vi "RIB - eSTOP 1.vi"(0 "Limits File Path":path, 5 "Results File Path":path, 11 "error in":errorcluster) -> (15 "error out":errorcluster)   [LabVIEW 2024]
doc: "Template test"
uses:
  <vilib>/addons/_JKI Toolkits/State Machine/_JKI_lib_State_Machine.llb/Select State(s)_err__jki_lib_state_machine.vi
  <vilib>/addons/_JKI Toolkits/State Machine/_JKI_lib_State_Machine.llb/Select State(s)_bool__jki_lib_state_machine.vi
  <vilib>/addons/_JKI Toolkits/State Machine/_JKI_lib_State_Machine.llb/Periodic Trigger__ogtk__JKI-SM__jki_lib_state_machine.vi
  <userlib>/_OpenG.lib/file/file.llb/Strip Path Extension - String__ogtk.vi
  <vilib>/Utility/file.llb/Read Delimited Spreadsheet (string).vi
  <userlib>/_OpenG.lib/file/file.llb/openg_file.lvlib
  <userlib>/_OpenG.lib/appcontrol/appcontrol.llb/openg_application_control.lvlib
  <userlib>/_OpenG.lib/time/time.llb/openg_time.lvlib
  <vilib>/Utility/file.llb/Write Delimited Spreadsheet (string).vi
panel:
  out "UDP Read Bar 2":dbl(slide) scale=0.0..10.0
  out "UDP Read Bar":dbl(slide) scale=0.0..10.0
  out "eSTOP 1 Test":bool
  out "eSTOP 1 Error Test":bool
  in  "eSTOP 1 Error Test":string
  in  "eSTOP 1 Test":string
  in  "connection ID":refnum<k16>
  out "Results Data Array":string[][](array[string])
  in  "handle out":u64
  in  "Exit":bool
  # "eSTOP 1 Test"
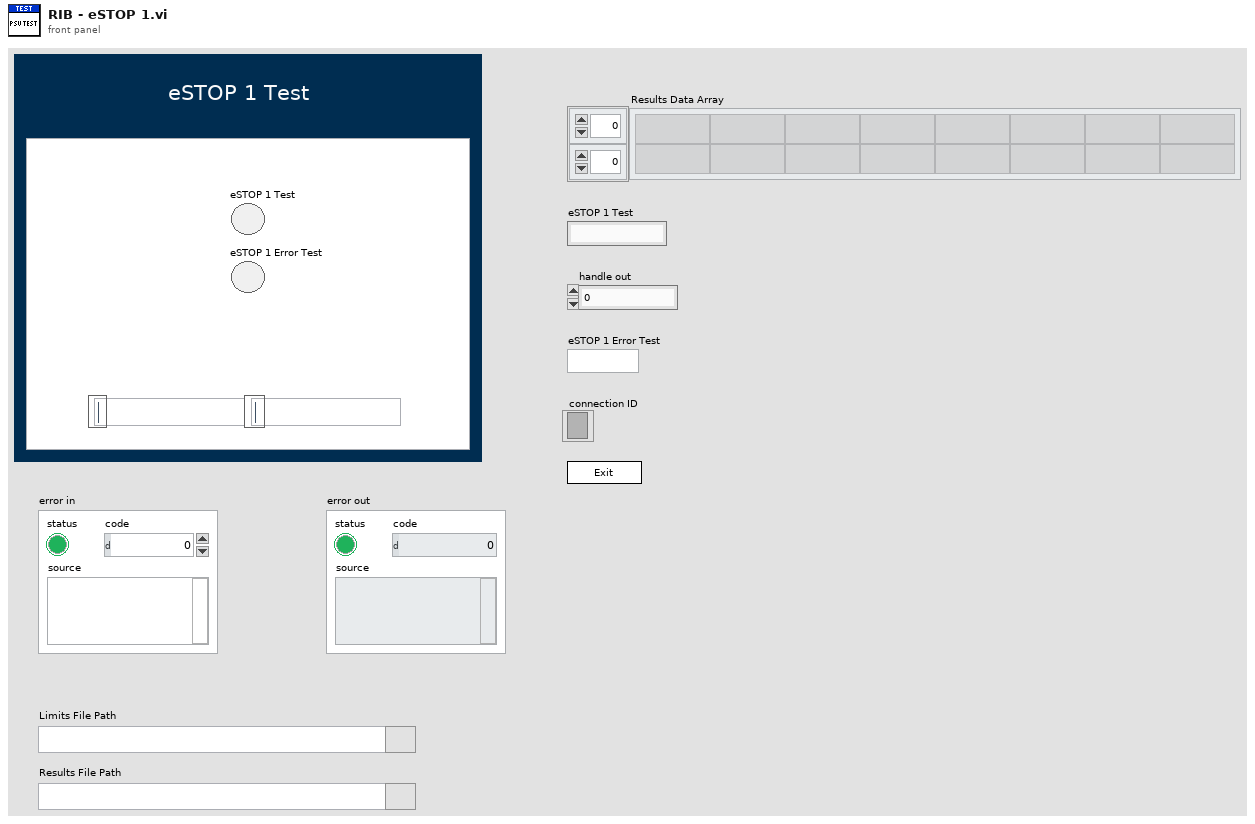
[diagram p1: front panel]
types:
  T1 = enum32{"Invalid", "Standard", "Closed", "Hidden", "Minimized", "Maximized"}
  T2 = enum32{"invalid app kind", "Development System", "Run Time System", "Student Edition", "Embedded LabVIEW", "Evaluation", "Custom"}
  T3 = typedef "FGV - Enum" = enum16{"Cleanup", "Get Data", "Open UDP", "Initialise DAQ", "Initialise I2C"}
  T4 = enum16{"Start Timer", "Get Time", "Pause", "Unpause"}
  T5 = cluster{"Core":cluster{"Current VI Reference":refnum<vi>, "Close Panel on Exit?":bool}, "Limits File Path":path, "Test Limits":string[][], "Results Data Array":string[][], "Results File Path":path, "Voltage":dbl, "connection ID":refnum<k16>, "handle out":u64, "eSTOP 1 Test":string, "eSTOP 1 Error Test":string}
  T6 = cluster{"Current VI Reference":refnum<vi>, "Close Panel on Exit?":bool}
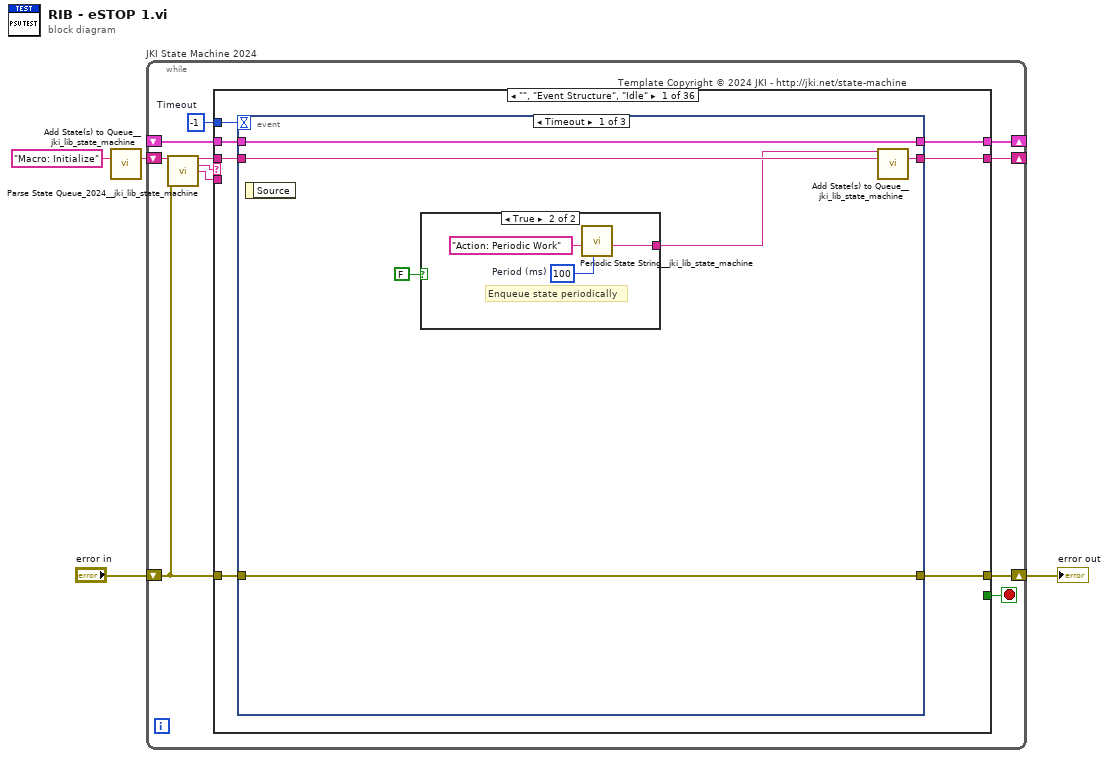
[diagram p0: block diagram]
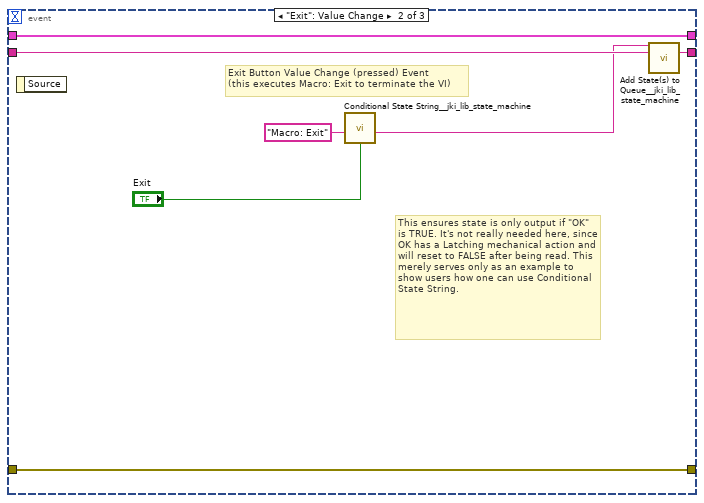
[diagram p3: hidden frame]
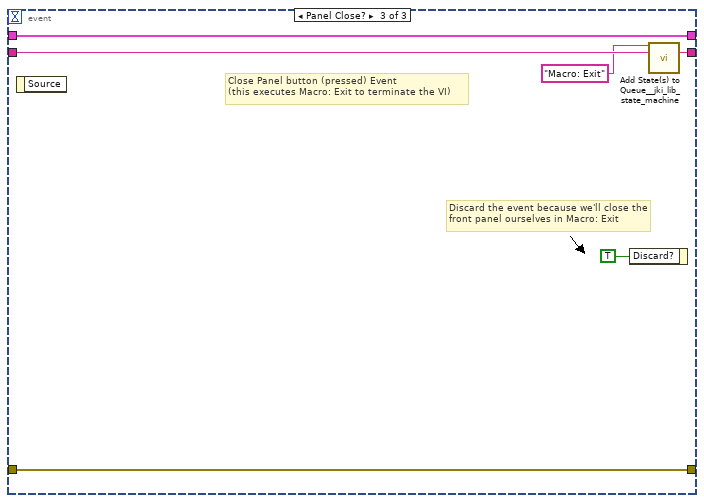
[diagram p4: hidden frame]
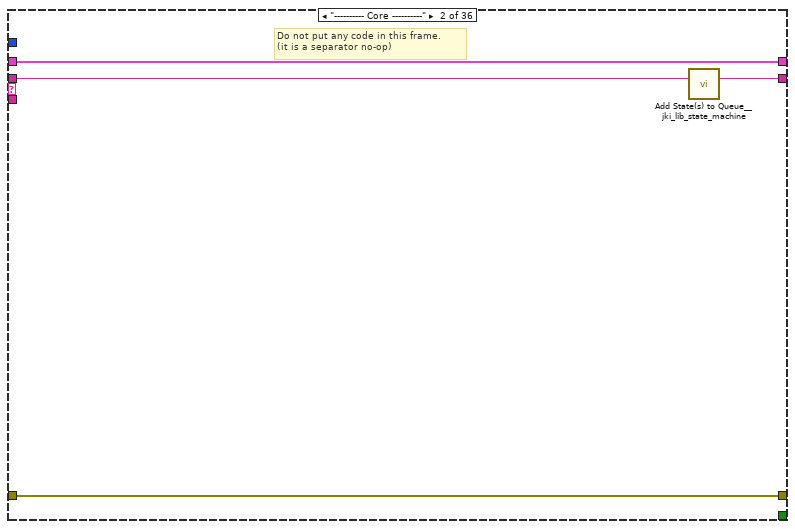
[diagram p5: hidden frame]
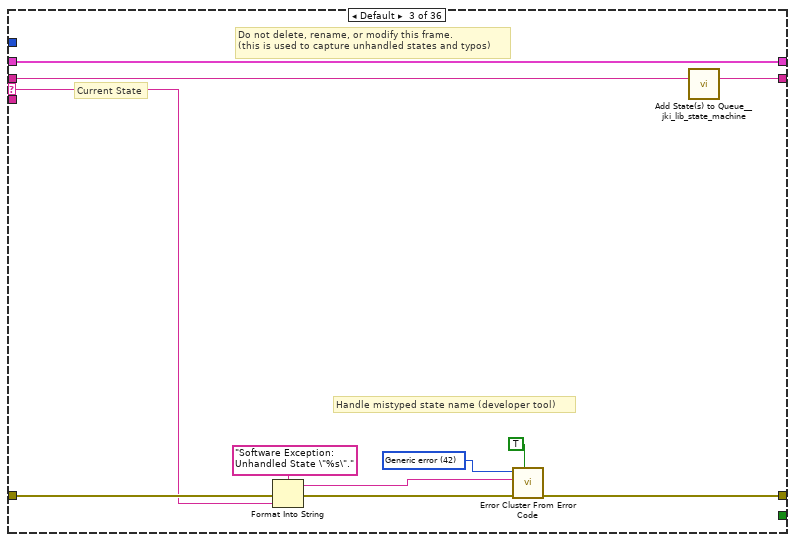
[diagram p6: hidden frame]
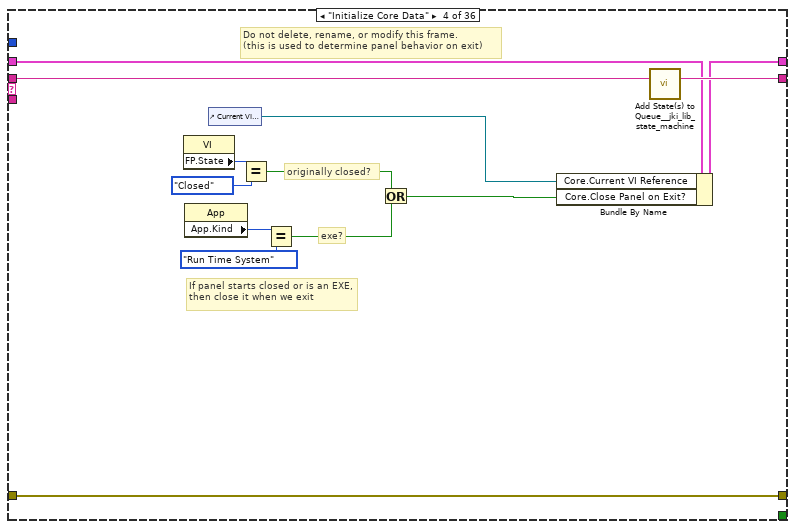
[diagram p7: hidden frame]
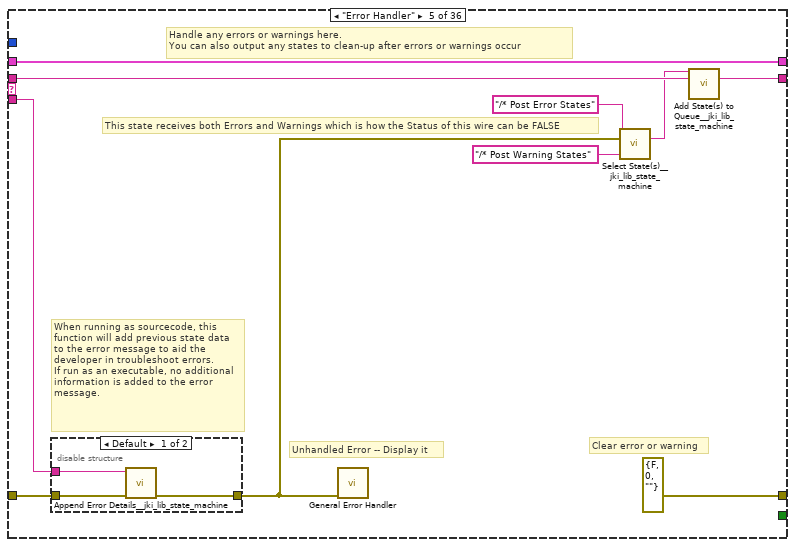
[diagram p8: hidden frame]
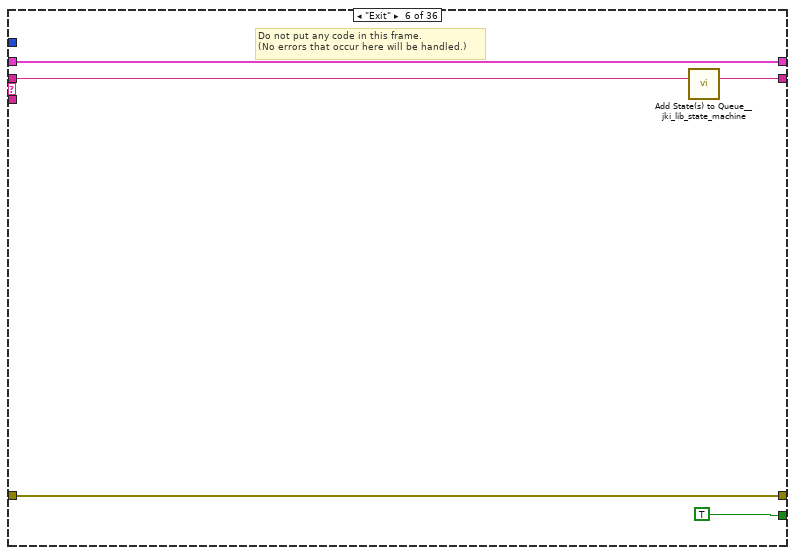
[diagram p10: hidden frame]
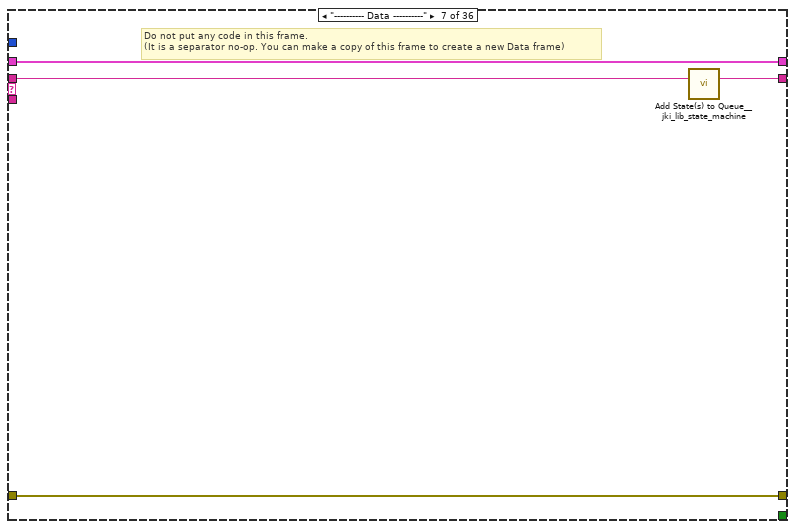
[diagram p11: hidden frame]
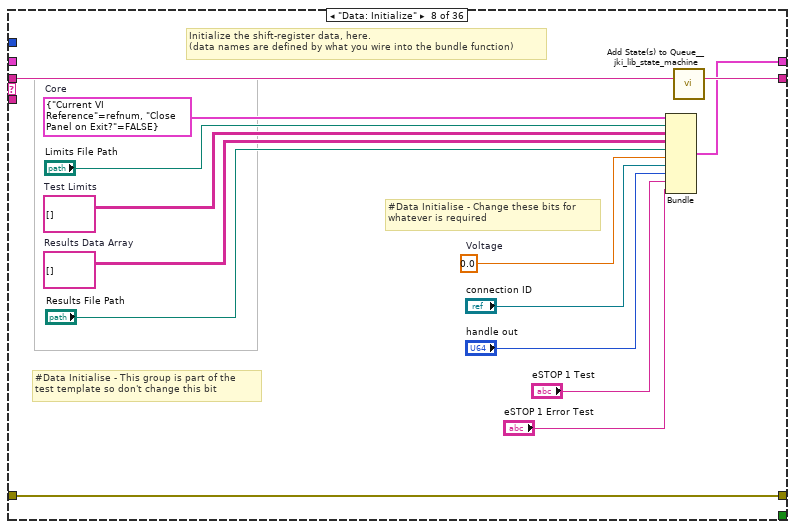
[diagram p12: hidden frame]
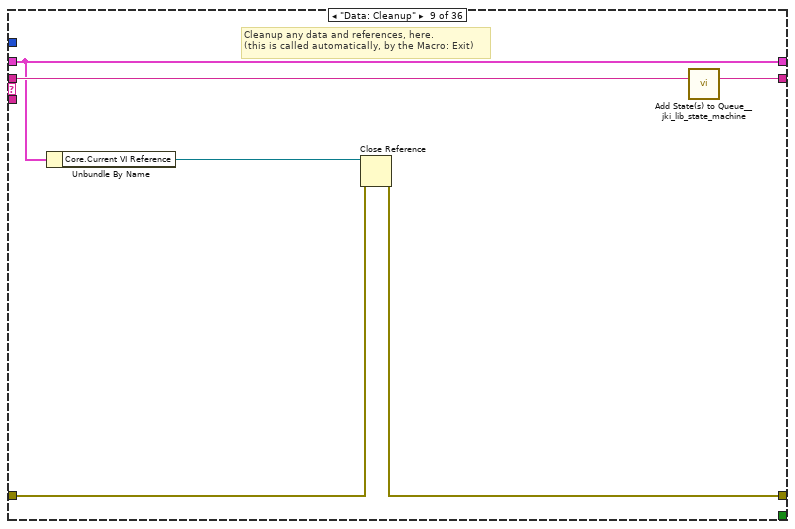
[diagram p13: hidden frame]
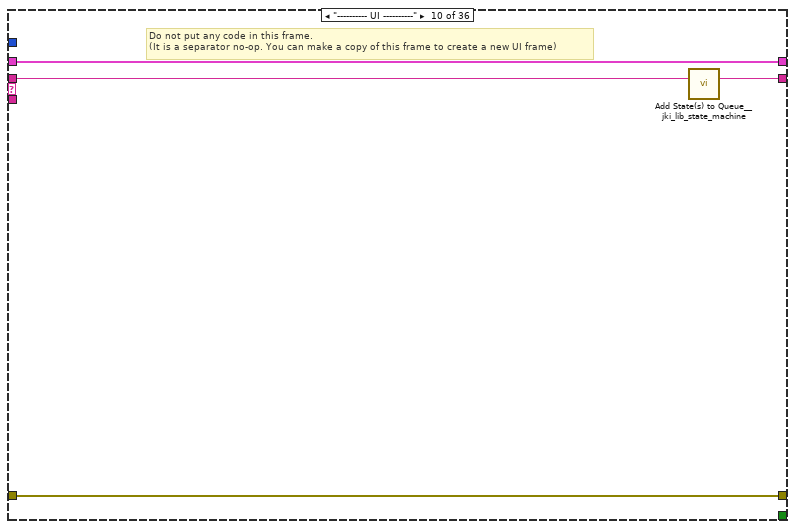
[diagram p14: hidden frame]
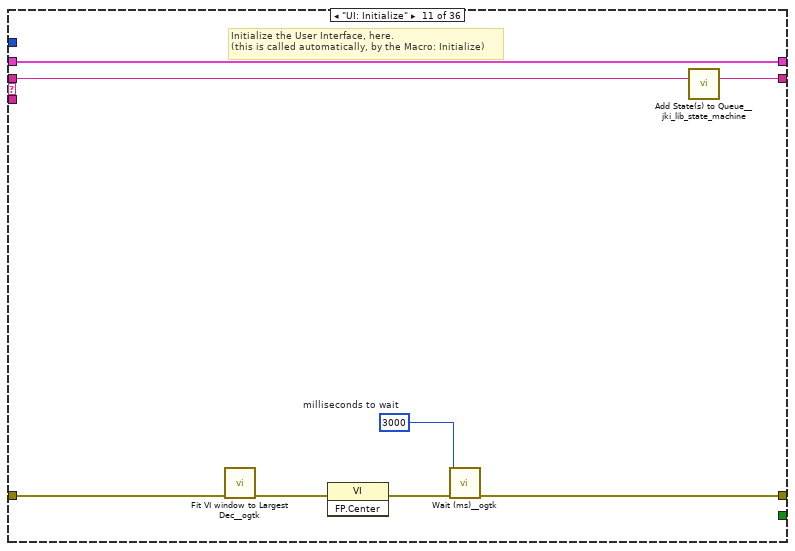
[diagram p15: hidden frame]
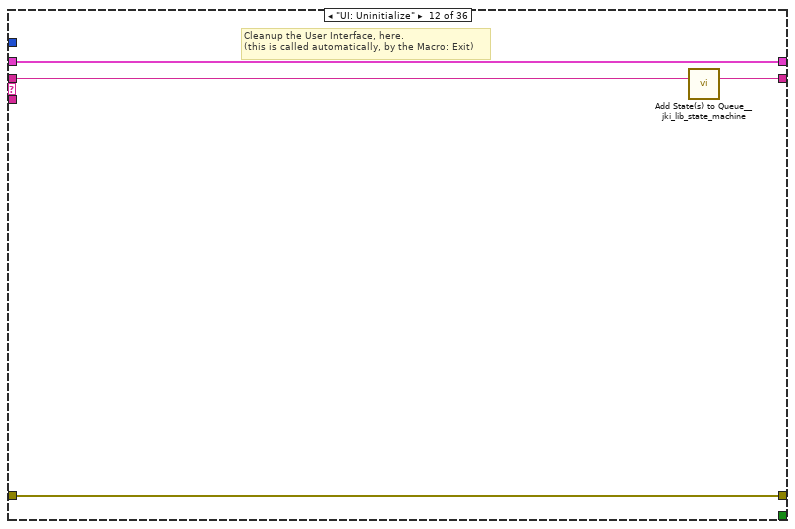
[diagram p16: hidden frame]
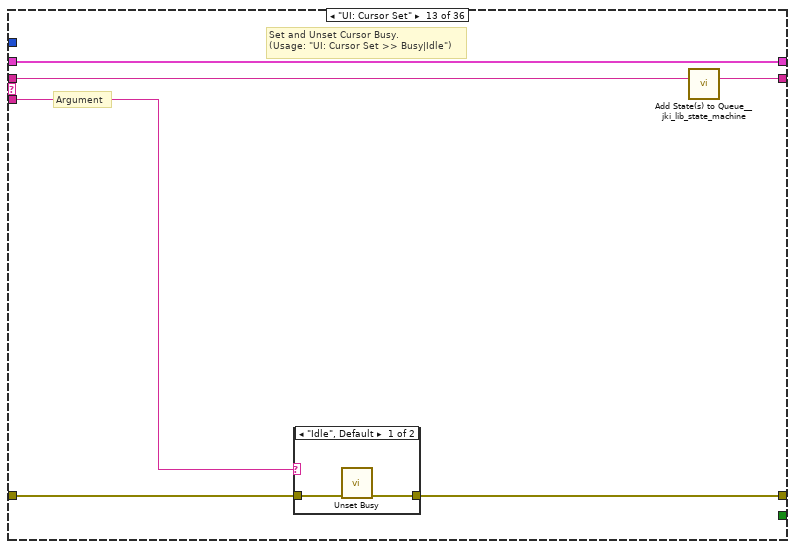
[diagram p17: hidden frame]
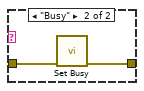
[diagram p18: hidden frame]
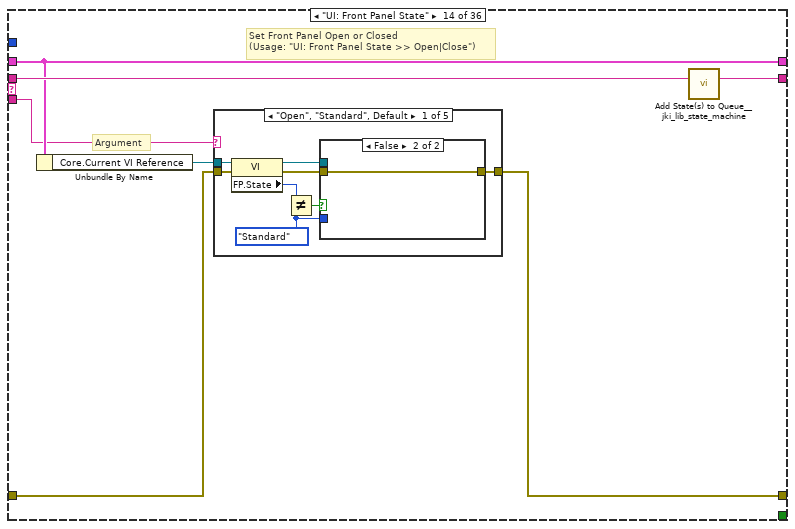
[diagram p19: hidden frame]
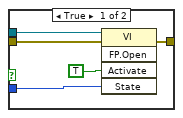
[diagram p20: hidden frame]
diagram:
  n1 = call <vilib>:"Add State(s) to Queue__jki_lib_state_machine.vi"("State(s) in (\"\")"="Macro: Initialize") -> ("States Out"=w4:string)  [unwired: 14 in]
  n2 = while "JKI State Machine 2024" {
    shift-right: [w8] -> _
    shift-left: _ -> [w7]
    shift-right: [w11] -> w1
    shift-left: "error in" -> [w5]
    shift-right: [w10] -> _
    shift-left: w4 -> [w12]
    stop <- w9 stop-if-true
    w6 = -1  # Timeout
    # "Template Copyright © 2024 JKI - http://jki.net/state-machine"
    n3 = call <vilib>:"Parse State Queue_2024__jki_lib_state_machine.vi"("State Queue"=w12, "Error In (no error)"=w5) -> ("Remaining States"=w14:string, "Current State"=w15:string, "Arguments"=w13:string)  [unwired: 11 in]
    n4 = case shown="\"\", \"Event Structure\", \"Idle\"" w15 {
      selector: w15 -> [_ _ w49 _ _ _ _ _ _ _ _ _ _ _ _ _ _ _ _ _ _ _ _ _ _ _ _ _ _ _ _ _ _ _ _ _]
      tunnel: w14 -> [w22 w48 w53 w72 w82 w91 w95 w109 w115 w119 w127 w131 w137 w148 w217 w222 w227 w232 w241 w245 w258 w275 w288 w292 w301 w305 w314 w324 w335 w344 w370 w380 w406 w418 w430 w439]
      tunnel: w13 -> [_ _ _ _ w77 _ _ _ _ _ _ _ w132 w142 _ _ _ _ _ _ _ _ _ _ _ _ _ _ _ _ _ _ _ _ _ _]
      tunnel: w7 -> [w20 w45 w51 w65 w79 w89 w92 _ w110 w116 w125 w129 w135 w144 w214 w219 w224 w229 w239 w242 w248 w267 w280 w289 w297 w302 w312 w322 w333 w338 w350 w374 w386 w416 w428 w432]
      tunnel: [w19 w46 w55 w69 errorcluster {"status"=FALSE, "code"=0, "source"=""} ("error out") w88 w93 w106 w111 w117 w123 w128 w133 w145 w215 w220 w225 w230 w236 w243 w254 w272 w285 w290 w299 w303 w309 w315 w326 w337 w348 w373 w384 w410 w422 w434] -> w11
      tunnel: w5 -> [w16 w46 w54 w69 w78 w88 w93 w106 w112 w117 w124 w128 w134 w146 w215 w220 w225 w230 w236 w243 w253 w271 w284 w290 w298 w303 w310 w316 w327 w341 w351 w377 w387 w411 w423 w433]
      tunnel: [w21 w47 w52 w71 w81 w90 w94 w108 w114 w118 w126 w130 w136 w147 w216 w221 w226 w231 w240 w244 w257 w274 w287 w291 w300 w304 w313 w323 w334 w343 w369 w379 w405 w417 w429 w438] -> w10
      tunnel: [_ _ _ _ _ TRUE _ _ _ _ _ _ _ _ _ _ _ _ _ _ _ _ _ _ _ _ _ _ _ _ _ _ _ _ _ _] -> w9
      tunnel: [w18 w45 w51 w70 w79 w89 w92 w107 w110 w116 w125 w129 w135 w144 w214 w219 w224 w229 w239 w242 w247 w266 w279 w289 w297 w302 w311 w322 w333 w336 w368 w372 w404 w416 w428 w431] -> w8
      tunnel: w6 -> [w17 _ _ _ _ _ _ _ _ _ _ _ _ _ _ _ _ _ _ _ _ _ _ _ _ _ _ _ _ _ _ _ _ _ _ _]
      frame "", "Event Structure", "Idle" {
        n5 = event shown="[0] Timeout" {
          selector: _ -> [_ _ _]
          dyn-events: _ -> [_ _ _]
          timeout: w17 -> [_ _ _]
          tunnel: w22 -> [w28 w38 w44]
          tunnel: [w27 w37 w43] -> w21
          tunnel: w20 -> [w25 w35 w41]
          tunnel: [w26 w36 w42] -> w19
          tunnel: w16 -> [w26 w36 w42]
          tunnel: [w25 w35 w41] -> w18
          event Timeout {
            n6 = event-data() -> ()  [unwired: 1 in, 1 out]
            n7 = case shown="True" FALSE {
              tunnel: [_ w31] -> w24
              frame False {
              }
              frame True {
                w29 = u32 100  # Period (ms)
                # "Enqueue state periodically"
                n8 = call <vilib>:"Periodic State String__jki_lib_state_machine.vi"("Period (ms)"=w29, "State"="Action: Periodic Work") -> ("State Out"=w31:string)  [unwired: 9 in]
              }
            }
            n9 = call <vilib>:"Add State(s) to Queue__jki_lib_state_machine.vi"("State(s) in Front (\"\")"=w24, "State(s) in (\"\")"=w28) -> ("States Out"=w27:string)  [unwired: 13 in]
          }
          event "Exit": Value Change {
            # "This ensures state is only output if \"OK\" is TRUE. It's not really needed here, since OK has a Latching mechanical action and will reset to FALSE after being read. This merely serves only as an example to show users how one can use Conditional State String."
            # "Exit Button Value Change (pressed) Event\n(this executes Macro: Exit to terminate the VI)"
            n10 = event-data() -> ()  [unwired: 1 in, 1 out]
            n11 = call <vilib>:"Conditional State String__jki_lib_state_machine.vi"("Do State(s)?"="Exit", "State"="Macro: Exit") -> ("State Out"=w32:string)  [unwired: 7 in]
            n12 = call <vilib>:"Add State(s) to Queue__jki_lib_state_machine.vi"("State(s) in Front (\"\")"=w32, "State(s) in (\"\")"=w38) -> ("States Out"=w37:string)  [unwired: 13 in]
          }
          event Panel Close? {
            # "Discard the event because we'll close the front panel ourselves in Macro: Exit"
            # "Close Panel button (pressed) Event\n(this executes Macro: Exit to terminate the VI)"
            n13 = event-data() -> ()  [unwired: 1 in, 1 out]
            n14 = event-data("Discard?"=TRUE) -> ()  [unwired: 1 in, 1 out]
            n15 = call <vilib>:"Add State(s) to Queue__jki_lib_state_machine.vi"("State(s) in Front (\"\")"="Macro: Exit", "State(s) in (\"\")"=w44) -> ("States Out"=w43:string)  [unwired: 13 in]
          }
        }
      }
      frame "---------- Core ----------" {
        # "Do not put any code in this frame.\n(it is a separator no-op)"
        n16 = call <vilib>:"Add State(s) to Queue__jki_lib_state_machine.vi"("State(s) in (\"\")"=w48) -> ("States Out"=w47:string)  [unwired: 14 in]
      }
      frame Default {
        w58 = 42 items=["No error", "Argument error", "Memory is full", "Out of zone", "End of file", "File already open", "Generic file I/O error", "File not found", "File permission error", "Disk is full", "Duplicate path", "Too many files open", "System feature not enabled", "Resource file not found", "Cannot add resource", "Resource not found", "Image not found", "Image memory error", "Pen does not exist", "Config type invalid", "Config token not found", "Config parse error", "Config memory error", "Bad external code format", "Bad external code offset", "External code not present", "Null window", "Destroy window error", "Null menu", "Print aborted", "Bad print record", "Print driver error", "Windows error during printing", "Memory error during printing", "Print dialog error", "Generic print error", "Invalid device refnum", "Device not found", "Device parameter error", "Device unit error", "Cannot open device", "Device call aborted", "Generic error", "Cancelled by user", "Object ID too low", "Object ID too high", "Object not in heap", "Unknown heap", "Unknown object (invalid DefProc)", "Unknown object (DefProc not in table)", "Message out of range", "Invalid (null) method", "Unknown message", "Manager call not supported", "Bad address", "Network operation in progress", "Network operation timed out", "Connection is busy", "Network attribute not supported", "Network error", "Address in use", "System out of memory", "Connection aborted", "Connection refused", "Not connected", "Already connected", "Connection closed", "Initialization error (interapplication manager)", "Bad occurrence", "Wait on unbound occurrence handler", "Occurrence queue overflow", "Datalog type conflict", "Unused", "Unrecognized type (interapplication manager)", "Memory corrupt", "Failed to make temporary DLL", "Old CIN version", "Drag socket not found", "Failed to load drop-object", "Failed to register OLE object", "Failed to release OLE object", "Format specifier type mismatch", "Unknown format specifier", "Too few format specifiers", "Too many format specifiers", "Scan failed", "Newer CIN version", "Error converting to variant", "Runtime menu error", "Password tampered", "Variant attribute not found", "Incompatible variant data type", "Event data is not available", "Event Store is not present", "Occurrence is not found", "Event Queue is not created", "Event info is not available", "Refnum passed is NULL", "Error retrieving Class GUID", "Error retrieving CoClass GUID", "Error retrieving TypeLib GUID.", "Bad built application magic bytes.", "Specific driver is different from the specific driver associated with the Logical Name.", "There is no session opened to the class driver.", "Max Error", "MAX - Error with config objects", "MAX - Error loading configuration", "MAX - Group not supported"]
        # "Current State"
        # "Do not delete, rename, or modify this frame.\n(this is used to capture unhandled states and typos)"
        # "Handle mistyped state name (developer tool)"
        n17 = Format Into String(format string="Software Exception: Unhandled State \"%s\"." ("message"), error in=w54, w49) -> (resulting string=w57:string, error out=w56:errorcluster)  [unwired: 1 in]
        n18 = call <vilib>:"Error Cluster From Error Code.vi"("show call chain? (False)"=TRUE, "error in (no error)"=w56, "error message (\"\")"=w57, "error code (0)"=w58) -> ("error out"=w55:errorcluster)  [unwired: 5 in]
        n19 = call <vilib>:"Add State(s) to Queue__jki_lib_state_machine.vi"("State(s) in (\"\")"=w53) -> ("States Out"=w52:string)  [unwired: 14 in]
      }
      frame "Initialize Core Data" {
        # "Do not delete, rename, or modify this frame.\n(this is used to determine panel behavior on exit)"
        # "originally closed?"
        # "exe?"
        # "If panel starts closed or is an EXE, then close it when we exit"
        n20 = property class="VI"() -> ("FP.State"=w62:T1)  [unwired: 2 in, 2 out]
        n21 = property class="App"() -> ("App.Kind"=w68:T2)  [unwired: 2 in, 2 out]
        n22 = control-ref of="Current VI Reference"() -> (w63:refnum<vi>)
        n23 = Equal?(x=w62, y=T1."Closed" ("Front Panel Window:State")) -> (x = y?=w60:bool)
        n24 = Equal?(x=w68, y=T2."Run Time System" ("Application:Kind")) -> (x = y?=w66:bool)
        n25 = Or(x=w60, y=w66) -> (x .or. y?=w64:bool)
        n26 = Bundle By Name(cluster=w65, "Core.Current VI Reference"=w63, "Core.Close Panel on Exit?"=w64) -> (w70:T5)
        n27 = call <vilib>:"Add State(s) to Queue__jki_lib_state_machine.vi"("State(s) in (\"\")"=w72) -> ("States Out"=w71:string)  [unwired: 14 in]
      }
      frame "Error Handler" {
        # "When running as sourcecode, this function will add previous state data to the error message to aid the developer in troubleshoot errors.\nIf run as an executable, no additional information is added to the error message."
        # "This state receives both Errors and Warnings which is how the Status of this wire can be FALSE"
        # "Unhandled Error -- Display it"
        # "Handle any errors or warnings here.\nYou can also output any states to clean-up after errors or warnings occur"
        # "Clear error or warning"
        n28 = disable-structure shown="Default" {
          disable-tunnel: w78 -> [w85 w86]
          disable-tunnel: w77 -> [w84 _]
          disable-tunnel: [w83 w86] -> w76
          frame condition #0 (active) {
            n29 = call <vilib>:"Append Error Details__jki_lib_state_machine.vi"("error in (no error)"=w85, "Previous State and Argument(s)"=w84) -> ("error out"=w83:errorcluster)  [unwired: 9 in]
          }
          frame condition #1 {
          }
        }
        n30 = call <vilib>:"General Error Handler.vi"("error in (no error)"=w76) -> ()  [unwired: 10 in, 5 out]
        n31 = call-poly <vilib>:"Select State(s)__jki_lib_state_machine.vi"("State(s) if True (\"\")"="/* Post Error States", "Select"=w76, "State(s) if False (\"\")"="/* Post Warning States") -> ("States Out"=w74:string)  [unwired: 12 in]
        n32 = call <vilib>:"Add State(s) to Queue__jki_lib_state_machine.vi"("State(s) in Front (\"\")"=w74, "State(s) in (\"\")"=w82) -> ("States Out"=w81:string)  [unwired: 13 in]
      }
      frame "Exit" {
        # "Do not put any code in this frame.\n(No errors that occur here will be handled.)"
        n33 = call <vilib>:"Add State(s) to Queue__jki_lib_state_machine.vi"("State(s) in (\"\")"=w91) -> ("States Out"=w90:string)  [unwired: 14 in]
      }
      frame "---------- Data ----------" {
        # "Do not put any code in this frame.\n(It is a separator no-op. You can make a copy of this frame to create a new Data frame)"
        n34 = call <vilib>:"Add State(s) to Queue__jki_lib_state_machine.vi"("State(s) in (\"\")"=w95) -> ("States Out"=w94:string)  [unwired: 14 in]
      }
      frame "Data: Initialize" {
        w100 = 0.0  # Voltage
        w102 = string[][] []  # Results Data Array
        w103 = string[][] []  # Test Limits
        w105 = T6 {"Current VI Reference"=refnum, "Close Panel on Exit?"=FALSE}  # Core
        # "#Data Initialise - Change these bits for\nwhatever is required"
        # "#Data Initialise - This group is part of the\ntest template so don't change this bit"
        # "Initialize the shift-register data, here.\n(data names are defined by what you wire into the bundle function)"
        n35 = Bundle("Core"=w105, "Limits File Path"="Limits File Path", "Test Limits"=w103, "Results Data Array"=w102, "Results File Path"="Results File Path", "Voltage"=w100, "connection ID"="connection ID", "handle out"="handle out", "eSTOP 1 Test"="eSTOP 1 Test", "eSTOP 1 Error Test"="eSTOP 1 Error Test") -> (w107:T5)  [unwired: 1 in]
        n36 = call <vilib>:"Add State(s) to Queue__jki_lib_state_machine.vi"("State(s) in (\"\")"=w109) -> ("States Out"=w108:string)  [unwired: 14 in]
      }
      frame "Data: Cleanup" {
        # "Cleanup any data and references, here.\n(this is called automatically, by the Macro: Exit)"
        n37 = Unbundle By Name(w110) -> ("Core.Current VI Reference"=w113:refnum<vi>)
        n38 = Close Reference(reference=w113, error in (no error)=w112) -> (error out=w111:errorcluster)
        n39 = call <vilib>:"Add State(s) to Queue__jki_lib_state_machine.vi"("State(s) in (\"\")"=w115) -> ("States Out"=w114:string)  [unwired: 14 in]
      }
      frame "---------- UI ----------" {
        # "Do not put any code in this frame.\n(It is a separator no-op. You can make a copy of this frame to create a new UI frame)"
        n40 = call <vilib>:"Add State(s) to Queue__jki_lib_state_machine.vi"("State(s) in (\"\")"=w119) -> ("States Out"=w118:string)  [unwired: 14 in]
      }
      frame "UI: Initialize" {
        w122 = u32 3000  # milliseconds to wait
        # "Initialize the User Interface, here.\n(this is called automatically, by the Macro: Initialize)"
        n41 = call <userlib>:"Fit VI window to Largest Dec__ogtk.vi"("error in (no error)"=w124) -> ("error out"=w120:errorcluster)  [unwired: 5 in, 1 out]
        n42 = invoke class="VI" method="FP.Center"(error in=w120) -> (error out=w121:errorcluster)  [unwired: 2 in, 2 out]
        n43 = call <userlib>:"Wait (ms)__ogtk.vi"("error in (no error)"=w121, "milliseconds to wait"=w122) -> ("error out"=w123:errorcluster)  [unwired: 8 in, 1 out]
        n44 = call <vilib>:"Add State(s) to Queue__jki_lib_state_machine.vi"("State(s) in (\"\")"=w127) -> ("States Out"=w126:string)  [unwired: 14 in]
      }
      frame "UI: Uninitialize" {
        # "Cleanup the User Interface, here.\n(this is called automatically, by the Macro: Exit)"
        n45 = call <vilib>:"Add State(s) to Queue__jki_lib_state_machine.vi"("State(s) in (\"\")"=w131) -> ("States Out"=w130:string)  [unwired: 14 in]
      }
      frame "UI: Cursor Set" {
        # "Argument"
        # "Set and Unset Cursor Busy.\n(Usage: \"UI: Cursor Set >> Busy|Idle\")"
        n46 = case shown="\"Idle\", Default" w132 {
          tunnel: w134 -> [w139 w141]
          tunnel: [w138 w140] -> w133
          frame "Idle", Default {
            n47 = call <vilib>:"Unset Busy.vi"("error in (no error)"=w139) -> ("error out"=w138:errorcluster)  [unwired: 10 in]
          }
          frame "Busy" {
            n48 = call <vilib>:"Set Busy.vi"("error in (no error)"=w141) -> ("error out"=w140:errorcluster)  [unwired: 9 in, 1 out]
          }
        }
        n49 = call <vilib>:"Add State(s) to Queue__jki_lib_state_machine.vi"("State(s) in (\"\")"=w137) -> ("States Out"=w136:string)  [unwired: 14 in]
      }
      frame "UI: Front Panel State" {
        # "Argument"
        # "Set Front Panel Open or Closed\n(Usage: \"UI: Front Panel State >> Open|Close\")"
        n50 = Unbundle By Name(w144) -> ("Core.Current VI Reference"=w143:refnum<vi>)
        n51 = case shown="\"Open\", \"Standard\", Default" w142 {
          tunnel: w146 -> [w154 w169 w180 w193 w206]
          tunnel: [w156 w170 w182 w195 w208] -> w145
          tunnel: w143 -> [w155 w167 w181 w194 w207]
          frame "Open", "Standard", Default {
            w149 = T1."Standard" ("State")
            n52 = property class="VI"(reference=w155, error in=w154) -> (reference out=w152:refnum<vi>, error out=w153:errorcluster, "FP.State"=w151:T1)
            n53 = Not Equal?(x=w151, y=w149) -> (x != y?=w150:bool)
            n54 = case shown="False" w150 {
              tunnel: [w160 w162] -> w156
              tunnel: w153 -> [w159 w162]
              tunnel: w152 -> [w158 _]
              tunnel: w149 -> [w157 _]
              frame True {
                n55 = invoke class="VI" method="FP.Open"(reference=w158, error in=w159, "Activate"=TRUE, "State"=w157) -> (error out=w160:errorcluster)  [unwired: 1 in, 4 out]
              }
              frame False {
              }
            }
          }
          frame "Close", "Closed" {
            n56 = property class="VI"(reference=w167, error in=w169) -> (reference out=w166:refnum<vi>, error out=w168:errorcluster, "FP.State"=w164:T1)
            n57 = Not Equal?(x=w164, y=T1."Closed" ("Front Panel Window:State")) -> (x != y?=w163:bool)
            n58 = case shown="True" w163 {
              tunnel: [w171 w174] -> w170
              tunnel: w168 -> [w171 w173]
              tunnel: w166 -> [_ w172]
              frame False {
              }
              frame True {
                n59 = invoke class="VI" method="FP.Close"(reference=w172, error in=w173) -> (error out=w174:errorcluster)  [unwired: 1 in, 2 out]
              }
            }
          }
          frame "Hidden", "Hide" {
            w175 = T1."Hidden" ("State")
            n60 = property class="VI"(reference=w181, error in=w180) -> (reference out=w178:refnum<vi>, error out=w179:errorcluster, "FP.State"=w177:T1)
            n61 = Not Equal?(x=w177, y=w175) -> (x != y?=w176:bool)
            n62 = case shown="True" w176 {
              tunnel: [w186 w187] -> w182
              tunnel: w179 -> [w185 w187]
              tunnel: w178 -> [w184 _]
              tunnel: w175 -> [w183 _]
              frame True {
                n63 = invoke class="VI" method="FP.Open"(reference=w184, error in=w185, "State"=w183) -> (error out=w186:errorcluster)  [unwired: 2 in, 4 out]
              }
              frame False {
              }
            }
          }
          frame "Minimize", "Minimized" {
            w188 = T1."Minimized" ("State")
            n64 = property class="VI"(reference=w194, error in=w193) -> (reference out=w191:refnum<vi>, error out=w192:errorcluster, "FP.State"=w190:T1)
            n65 = Not Equal?(x=w190, y=w188) -> (x != y?=w189:bool)
            n66 = case shown="True" w189 {
              tunnel: [w199 w200] -> w195
              tunnel: w192 -> [w198 w200]
              tunnel: w191 -> [w197 _]
              tunnel: w188 -> [w196 _]
              frame True {
                n67 = invoke class="VI" method="FP.Open"(reference=w197, error in=w198, "State"=w196) -> (error out=w199:errorcluster)  [unwired: 2 in, 4 out]
              }
              frame False {
              }
            }
          }
          frame "Maximize", "Maximized" {
            w201 = T1."Maximized" ("State")
            n68 = property class="VI"(reference=w207, error in=w206) -> (reference out=w204:refnum<vi>, error out=w205:errorcluster, "FP.State"=w203:T1)
            n69 = Not Equal?(x=w203, y=w201) -> (x != y?=w202:bool)
            n70 = case shown="True" w202 {
              tunnel: [w212 w213] -> w208
              tunnel: w205 -> [w211 w213]
              tunnel: w204 -> [w210 _]
              tunnel: w201 -> [w209 _]
              frame True {
                n71 = invoke class="VI" method="FP.Open"(reference=w210, error in=w211, "State"=w209) -> (error out=w212:errorcluster)  [unwired: 2 in, 4 out]
              }
              frame False {
              }
            }
          }
        }
        n72 = call <vilib>:"Add State(s) to Queue__jki_lib_state_machine.vi"("State(s) in (\"\")"=w148) -> ("States Out"=w147:string)  [unwired: 14 in]
      }
      frame "---------- Macro ----------" {
        # "Do not put any code in this frame.\n(It is a separator no-op. You can make a copy of this frame to create a new Macro frame)"
        n73 = call <vilib>:"Add State(s) to Queue__jki_lib_state_machine.vi"("State(s) in (\"\")"=w217) -> ("States Out"=w216:string)  [unwired: 14 in]
      }
      frame "Macro: Initialize" {
        # "Initialization Macro\n(This is called once, when the VI starts)"
        n74 = call <vilib>:"Add State(s) to Queue__jki_lib_state_machine.vi"("State(s) in Front (\"\")"="Data: Initialize\nInitialize Core Data\nUI: Initialize\nUI: Front Panel State >> Open\neSTOP1 Test: Initialise\nMacro: Test", "State(s) in (\"\")"=w222) -> ("States Out"=w221:string)  [unwired: 13 in]
      }
      frame "Macro: Test" {
        # "#Test Macro - Add the sequence \nfor measurments and limits testing here"
        n75 = call <vilib>:"Add State(s) to Queue__jki_lib_state_machine.vi"("State(s) in Front (\"\")"="Limits Test: Read Limits File\neSTOP1 Test: Start Timer\neSTOP1 Test: I2C Measurment\neSTOP1 Test: UDP Read", "State(s) in (\"\")"=w227) -> ("States Out"=w226:string)  [unwired: 13 in]
      }
      frame "Macro: Limits" {
        # "Do not put any code in this frame.\n(It is a separator no-op. You can make a copy of this frame to create a new Macro frame)"
        n76 = call <vilib>:"Add State(s) to Queue__jki_lib_state_machine.vi"("State(s) in Front (\"\")"="Limits Test: eSTOP 1 Test\nLimits Test: eSTOP 1 Error Test\nResults Data: Write Results Data\nMacro: Exit", "State(s) in (\"\")"=w232) -> ("States Out"=w231:string)  [unwired: 13 in]
      }
      frame "Macro: Exit" {
        # "Exit Macro\n(This is called once, when the VI exits)"
        n77 = Unbundle By Name(w239) -> ("Core.Close Panel on Exit?"=w234:bool)
        n78 = call <vilib>:"Conditional State String__jki_lib_state_machine.vi"("Do State(s)?"=w234, "State"="UI: Front Panel State >> Close") -> ("State Out"=w233:string)  [unwired: 7 in]
        n79 = call <vilib>:"Add State(s) to Queue__jki_lib_state_machine.vi"("State(s) in (\"\")"=w233, "State(s) at Back (\"\")"="eSTOP1 Test: Cleanup\nUI: Uninitialize\nData: Cleanup\nExit") -> ("States Out"=w237:string)  [unwired: 13 in]
        n80 = call <vilib>:"Add State(s) to Queue__jki_lib_state_machine.vi"("State(s) in Front (\"\")"=w237, "State(s) in (\"\")"=w241) -> ("States Out"=w240:string)  [unwired: 13 in]
      }
      frame "---------- Limits Test ----------" {
        # "Template Separator\n(You can make a copy of, or modify, this frame)"
        n81 = call <vilib>:"Add State(s) to Queue__jki_lib_state_machine.vi"("State(s) in (\"\")"=w245) -> ("States Out"=w244:string)  [unwired: 14 in]
      }
      frame "Limits Test: Read Limits File" {
        w251 = ","  # delimiter (\t)
        n82 = Unbundle By Name(w248) -> ("Limits File Path"=w252:path)
        n83 = Current VI's Path "Test Case Path"() -> (path=w256:path)
        n84 = call-poly <vilib>:"Read Delimited Spreadsheet.vi"("file path (dialog if empty)"=w252, "error in (no error)"=w253, "delimiter (\\t)"=w251) -> ("all rows"=w249:string[][], "error out"=w254:errorcluster)  [unwired: 7 in, 4 out]
        n85 = Strip Path(path=w256) -> (name=w255:string)  [unwired: 1 out]
        n86 = call-poly <userlib>:"Strip Path Extension__ogtk.vi"("path"=w255) -> ("root"=w250:string)  [unwired: 1 out]
        n87 = for {
          tunnel: w250 -> [w262]
          tunnel: w249 -> [w260] mode=indexing
          tunnel: [w260] -> w246 mode=indexing if=w259
          n88 = Index Array(array=w260) -> (element=w261:string)  [unwired: 1 in]
          n89 = Equal?(x=w262, y=w261) -> (x = y?=w259:bool)
        }
        n90 = Bundle By Name(cluster=w248, "Test Limits"=w246) -> (w247:T5)
        n91 = call <vilib>:"Add State(s) to Queue__jki_lib_state_machine.vi"("State(s) in (\"\")"=w258) -> ("States Out"=w257:string)  [unwired: 14 in]
      }
      frame "Limits Test: eSTOP 1 Test" {
        w268 = "eSTOP 1 Test"  # Sub Test Name
        # "Equal to F1?"
        # "#Limits Testing - Add the sub test name for\ntest included in limits file"
        n92 = Unbundle By Name(w267) -> ("Test Limits"=w269:string[][], "eSTOP 1 Test"=w273:string)
        n93 = Unbundle By Name(w267) -> ("Results Data Array"=w265:string[][])
        n94 = To Variant(anything=w273) -> (Variant=w270:variant)
        n95 = call "Process Results.vi"("error in (no error)"=w271, "Measurment"=w270, "Test Limits"=w269, "Sub Test Name"=w268) -> ("error out"=w272:errorcluster, "Results Data"=w264:string[])  [unwired: 6 in]
        n96 = Build Array (concatenate)(w265, w264) -> (w263:string[][])
        n97 = Bundle By Name(cluster=w267, "Results Data Array"=w263) -> (w266:T5)
        n98 = call <vilib>:"Add State(s) to Queue__jki_lib_state_machine.vi"("State(s) in (\"\")"=w275) -> ("States Out"=w274:string)  [unwired: 14 in]
      }
      frame "Limits Test: eSTOP 1 Error Test" {
        w281 = "eSTOP 1 Error Test"  # Sub Test Name
        # "Equal to FF ?"
        # "#Limits Testing - Add the sub test name for\ntest included in limits file"
        n99 = Unbundle By Name(w280) -> ("Test Limits"=w282:string[][], "eSTOP 1 Error Test"=w286:string)
        n100 = Unbundle By Name(w280) -> ("Results Data Array"=w278:string[][])
        n101 = To Variant(anything=w286) -> (Variant=w283:variant)
        n102 = call "Process Results.vi"("error in (no error)"=w284, "Measurment"=w283, "Test Limits"=w282, "Sub Test Name"=w281) -> ("error out"=w285:errorcluster, "Results Data"=w277:string[])  [unwired: 6 in]
        n103 = Build Array (concatenate)(w278, w277) -> (w276:string[][])
        n104 = Bundle By Name(cluster=w280, "Results Data Array"=w276) -> (w279:T5)
        n105 = call <vilib>:"Add State(s) to Queue__jki_lib_state_machine.vi"("State(s) in (\"\")"=w288) -> ("States Out"=w287:string)  [unwired: 14 in]
      }
      frame "---------- Results Data ----------" {
        # "Template Separator\n(You can make a copy of, or modify, this frame)"
        n106 = call <vilib>:"Add State(s) to Queue__jki_lib_state_machine.vi"("State(s) in (\"\")"=w292) -> ("States Out"=w291:string)  [unwired: 14 in]
      }
      frame "Results Data: Write Results Data" {
        w294 = ","  # delimiter (\t)
        w295 = TRUE  # append to file? (new file:F)
        n107 = Unbundle By Name(w297) -> ("Results File Path"=w296:path, "Results Data Array"=w293:string[][])
        "Results Data Array" <- w293
        n108 = call-poly <vilib>:"Write Delimited Spreadsheet.vi"("file path (dialog if empty)"=w296, "2D data"=w293, "append to file? (new file:F)"=w295, "error in (no error)"=w298, "delimiter (\\t)"=w294) -> ("error out"=w299:errorcluster)  [unwired: 9 in, 1 out]
        n109 = call <vilib>:"Add State(s) to Queue__jki_lib_state_machine.vi"("State(s) in (\"\")"=w301) -> ("States Out"=w300:string)  [unwired: 14 in]
      }
      frame "---------- eSTOP1 Test ----------" {
        # "Template Separator\n(You can make a copy of, or modify, this frame)"
        n110 = call <vilib>:"Add State(s) to Queue__jki_lib_state_machine.vi"("State(s) in (\"\")"=w305) -> ("States Out"=w304:string)  [unwired: 14 in]
      }
      frame "eSTOP1 Test: Initialise" {
        # "Measurement initialisation code goes here"
        n111 = call "FGV - Initialise.vi"("Enum"=FGV_-_Enum."Get Data", "Error In"=w310) -> ("connection ID"=w307:refnum<k16>, "Handle Out"=w306:u64, "Error Out"=w309:errorcluster)  [unwired: 10 in, 1 out]
        n112 = Bundle By Name(cluster=w312, "connection ID"=w307, "handle out"=w306) -> (w311:T5)
        n113 = call <vilib>:"Add State(s) to Queue__jki_lib_state_machine.vi"("State(s) in (\"\")"=w314) -> ("States Out"=w313:string)  [unwired: 14 in]
      }
      frame "eSTOP1 Test: Start Timer" {
        # "Start Timer and slide bar"
        # "Template Separator\n(You can make a copy of, or modify, this frame)"
        n114 = call "Timer.vi"("error in (no error)"=w316, "Enum"=T4."Start Timer") -> ("error out"=w320:errorcluster)  [unwired: 6 in, 3 out]
        n115 = property on="UDP Read Bar" class="Slide (strict)"(error in=w320, "Value"=0.0 ("Horizontal Pointer Slide"), "Scale.Maximum"=3.0 ("Target Time"), "Scale.Minimum"=0.0 ("Scale.Range:Minimum")) -> (error out=w315:errorcluster)  [unwired: 1 in, 1 out]
        n116 = call <vilib>:"Add State(s) to Queue__jki_lib_state_machine.vi"("State(s) in (\"\")"=w324) -> ("States Out"=w323:string)  [unwired: 14 in]
      }
      frame "eSTOP1 Test: Start Timer (Error)" {
        # "Template Separator\n(You can make a copy of, or modify, this frame)"
        n117 = call "Timer.vi"("error in (no error)"=w327, "Enum"=T4."Start Timer") -> ("error out"=w331:errorcluster)  [unwired: 6 in, 3 out]
        n118 = property on="UDP Read Bar 2" class="Slide (strict)"(error in=w331, "Value"=0.0 ("Horizontal Pointer Slide"), "Scale.Maximum"=3.0 ("Target Time"), "Scale.Minimum"=0.0 ("Scale.Range:Minimum")) -> (error out=w326:errorcluster)  [unwired: 1 in, 1 out]
        n119 = call <vilib>:"Add State(s) to Queue__jki_lib_state_machine.vi"("State(s) in Front (\"\")"="eSTOP1 Test: I2C Error Measurment" ("State(s) if True (\"\")"), "State(s) in (\"\")"=w335) -> ("States Out"=w334:string)  [unwired: 13 in]
      }
      frame "eSTOP1 Test: I2C Measurment" {
        # "switch realy - trigger estop 1"
        n120 = Unbundle By Name(w338) -> ("handle out"=w340:u64)
        n121 = call "PCA9525 - Estop 1.vi"("error in (no error)"=w341, "buffer"=u8[] [2, 86, 0], "handle"=w340) -> ("error out"=w337:errorcluster, "handle out"=w339:u64)  [unwired: 6 in, 1 out]
        n122 = Bundle By Name(cluster=w338, "handle out"=w339) -> (w336:T5)
        n123 = call <vilib>:"Add State(s) to Queue__jki_lib_state_machine.vi"("State(s) in (\"\")"=w344) -> ("States Out"=w343:string)  [unwired: 14 in]
      }
      frame "eSTOP1 Test: UDP Read" {
        # "Read UDP if equal to F1 then test complete if false timer is check if elapsed"
        n124 = Unbundle By Name(w350) -> ("connection ID"=w360:refnum<k16>)
        n125 = UDP Read(connection ID=w360, timeout ms (25000)=100, 8:w351) -> (data out=w345:string, error out=w349:errorcluster, 3:w359:refnum<k16>)  [unwired: 1 in, 2 out]
        n126 = String Subset(string=w345, offset (0)=81 ("offset (0) 2"), length (rest)=1 ("length (rest) 2")) -> (substring=w358:string)
        n127 = String To Byte Array(string=w358) -> (unsigned byte array=w367:u8[])
        n128 = Equal?(x=w358, y="ñ") -> (x = y?=→"eSTOP 1 Test":bool)
        n129 = Number To Hexadecimal String(2:w367) -> (0:w366:string[])  [unwired: 1 in]
        n130 = Index Array(array=w366, index=0) -> (element=w353:string)
        n131 = Equal?(x=w353, y="F1") -> (x = y?=w355:bool)
        n132 = Bundle By Name(cluster=w350, "connection ID"=w359, "eSTOP 1 Test"=w353) -> (w368:T5)
        n133 = call <vilib>:"Clear Errors.vi"("error in (no error)"=w349, "specific error code to clear (0: all)"=56) -> ("error out"=w348:errorcluster)  [unwired: 4 in, 1 out]
        n134 = call-poly <vilib>:"Select State(s)__jki_lib_state_machine.vi"("State(s) if True (\"\")"="eSTOP1 Test: Start Timer (Error)" ("State(s) if True (\"\")"), "Select"=w355, "State(s) if False (\"\")"="eSTOP1 Test: Elapsed Timer" ("State(s) if False (\"\")")) -> ("States Out"=w352:string)  [unwired: 12 in]
        n135 = call <vilib>:"Add State(s) to Queue__jki_lib_state_machine.vi"("State(s) in Front (\"\")"=w352, "State(s) in (\"\")"=w370) -> ("States Out"=w369:string)  [unwired: 13 in]
      }
      frame "eSTOP1 Test: I2C Error Measurment" {
        # "switch relay - force error"
        n136 = Unbundle By Name(w374) -> ("handle out"=w376:u64)
        n137 = call "PCA9525 - Estop 1.vi"("error in (no error)"=w377, "buffer"=u8[] [2, 3, 0], "handle"=w376) -> ("error out"=w373:errorcluster, "handle out"=w375:u64)  [unwired: 6 in, 1 out]
        n138 = Bundle By Name(cluster=w374, "handle out"=w375) -> (w372:T5)
        n139 = call <vilib>:"Add State(s) to Queue__jki_lib_state_machine.vi"("State(s) in Front (\"\")"="eSTOP1 Test: Error UDP Read" ("State(s) if True (\"\")"), "State(s) in (\"\")"=w380) -> ("States Out"=w379:string)  [unwired: 13 in]
      }
      frame "eSTOP1 Test: Error UDP Read" {
        # "Read UDP if equal to FF test complete if false check if timer has elapsed."
        n140 = Unbundle By Name(w386) -> ("connection ID"=w398:refnum<k16>)
        n141 = UDP Read(connection ID=w398, timeout ms (25000)=100, 8:w387) -> (data out=w403:string, error out=w385:errorcluster, 3:w397:refnum<k16>)  [unwired: 1 in, 2 out]
        n142 = String Subset(string=w403, offset (0)=81 ("offset (0) 2"), length (rest)=1 ("length (rest) 2")) -> (substring=w381:string)
        n143 = String To Byte Array(string=w381) -> (unsigned byte array=w396:u8[])
        n144 = Equal?(x=w381, y="ÿ") -> (x = y?=→"eSTOP 1 Error Test":bool)
        n145 = Number To Hexadecimal String(2:w396) -> (0:w395:string[])  [unwired: 1 in]
        n146 = Index Array(array=w395, index=0) -> (element=w389:string)
        n147 = Bundle By Name(cluster=w386, "connection ID"=w397, "eSTOP 1 Error Test"=w389) -> (w404:T5)
        n148 = Equal?(x=w389, y="FF") -> (x = y?=w393:bool)
        n149 = call <vilib>:"Clear Errors.vi"("error in (no error)"=w385, "specific error code to clear (0: all)"=56) -> ("error out"=w384:errorcluster)  [unwired: 4 in, 1 out]
        n150 = call-poly <vilib>:"Select State(s)__jki_lib_state_machine.vi"("State(s) if True (\"\")"="Macro: Limits" ("State(s) if True (\"\")"), "Select"=w393, "State(s) if False (\"\")"="eSTOP1 Test: Elapsed Timer (Error)" ("State(s) if False (\"\")")) -> ("States Out"=w388:string)  [unwired: 12 in]
        n151 = call <vilib>:"Add State(s) to Queue__jki_lib_state_machine.vi"("State(s) in Front (\"\")"=w388, "State(s) in (\"\")"=w406) -> ("States Out"=w405:string)  [unwired: 13 in]
      }
      frame "eSTOP1 Test: Elapsed Timer" {
        # "check if timer elapsed if true end of test if false UDP is read again,"
        # "Template Separator\n(You can make a copy of, or modify, this frame)"
        n152 = call "Timer.vi"("error in (no error)"=w411, "Target Time"=3.0, "Enum"=T4."Get Time") -> ("error out"=w410:errorcluster, "Time Elapsed?"=w412:bool, "Elapsed Time"=→"UDP Read Bar":dbl)  [unwired: 5 in, 1 out]
        n153 = call-poly <vilib>:"Select State(s)__jki_lib_state_machine.vi"("State(s) if True (\"\")"="eSTOP1 Test: Start Timer (Error)" ("State(s) if True (\"\")"), "Select"=w412, "State(s) if False (\"\")"="eSTOP1 Test: UDP Read" ("State(s) if False (\"\")")) -> ("States Out"=w409:string)  [unwired: 12 in]
        n154 = call <vilib>:"Add State(s) to Queue__jki_lib_state_machine.vi"("State(s) in Front (\"\")"=w409, "State(s) in (\"\")"=w418) -> ("States Out"=w417:string)  [unwired: 13 in]
      }
      frame "eSTOP1 Test: Elapsed Timer (Error)" {
        # "check if timer elapsed if true end of test if false UDP is read again,"
        # "Template Separator\n(You can make a copy of, or modify, this frame)"
        n155 = call "Timer.vi"("error in (no error)"=w423, "Target Time"=3.0, "Enum"=T4."Get Time") -> ("error out"=w422:errorcluster, "Time Elapsed?"=w424:bool, "Elapsed Time"=→"UDP Read Bar 2":dbl)  [unwired: 5 in, 1 out]
        n156 = call-poly <vilib>:"Select State(s)__jki_lib_state_machine.vi"("State(s) if True (\"\")"="Macro: Limits" ("State(s) if True (\"\")"), "Select"=w424, "State(s) if False (\"\")"="eSTOP1 Test: Error UDP Read" ("State(s) if False (\"\")")) -> ("States Out"=w421:string)  [unwired: 12 in]
        n157 = call <vilib>:"Add State(s) to Queue__jki_lib_state_machine.vi"("State(s) in Front (\"\")"=w421, "State(s) in (\"\")"=w430) -> ("States Out"=w429:string)  [unwired: 13 in]
      }
      frame "eSTOP1 Test: Cleanup" {
        # "Switch relays - back to Initialize state"
        # "Measurment cleanup code goes here"
        n158 = Unbundle By Name(w432) -> ("handle out"=w436:u64)
        n159 = call "PCA9525 - Estop 1.vi"("error in (no error)"=w433, "buffer"=u8[] [2, 85, 0], "handle"=w436) -> ("error out"=w434:errorcluster, "handle out"=w435:u64)  [unwired: 6 in, 1 out]
        n160 = Bundle By Name(cluster=w432, "handle out"=w435) -> (w431:T5)
        n161 = call <vilib>:"Add State(s) to Queue__jki_lib_state_machine.vi"("State(s) in (\"\")"=w439) -> ("States Out"=w438:string)  [unwired: 14 in]
      }
    }
  }
  "error out" <- w1
